vi "Create.vi"(5 "TestResultMock In":refnum<class "TestResultMock.lvclass">, 8 "error in (no error)":errorcluster) -> (0 "error out":errorcluster, 3 "TestResultMock":refnum<class "TestResultMock.lvclass">)   [LabVIEW 2019, in "TestSuiteTest.lvlib" / "Support.lvlib" / "TestResultMock.lvclass"]
uses:
  TestResultMock.lvclass
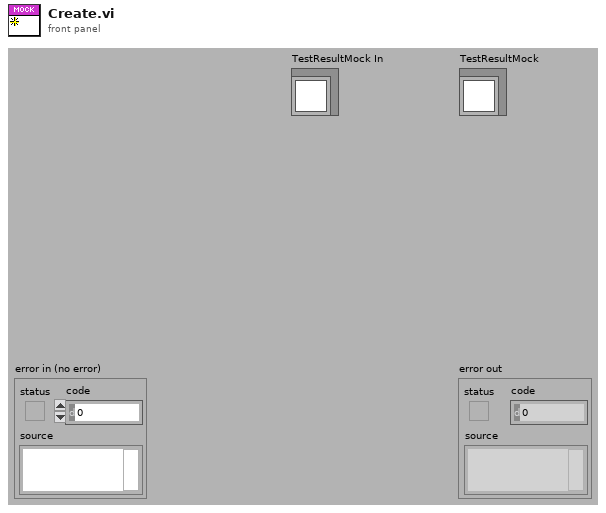
[diagram p1: front panel]
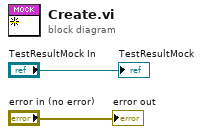
[diagram p0: block diagram]
diagram:
  "error out" <- "error in (no error)"
  "TestResultMock" <- "TestResultMock In"
